vi "fpga_8ch_Timestamping_BaselineCh_ov_debug.vi"(0 "Main clock":u32, 1 "Scheduler":u8, 2 "Baseline Ch":u8, 3 "Signal IN":T2, 4 "overflow":bool) -> (5 "Data available":T2, 6 "Timeouts Bundle":T1, 7 "Timestamp bundle":T3)   [LabVIEW 2011]
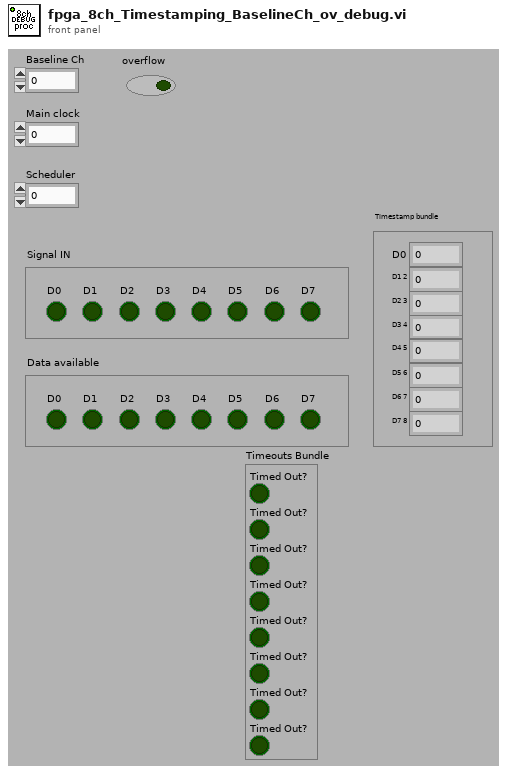
[diagram p1: front panel]
types:
  T1 = cluster{"Timed Out?":bool, "Timed Out?":bool, "Timed Out?":bool, "Timed Out?":bool, "Timed Out?":bool, "Timed Out?":bool, "Timed Out?":bool, "Timed Out?":bool}
  T2 = cluster{"D0":bool, "D1":bool, "D2":bool, "D3":bool, "D4":bool, "D5":bool, "D6":bool, "D7":bool}
  T3 = cluster{"D0":u32, "D1 2":u32, "D2 3":u32, "D3 4":u32, "D4 5":u32, "D5 6":u32, "D6 7":u32, "D7 8":u32}
  T4 = cluster{"Data Available":bool, "Data Available":bool, "Data Available":bool, "Data Available":bool, "Data Available":bool, "Data Available":bool, "Data Available":bool, "Data Available":bool}
  T5 = cluster{"32 bit Output":u32, "32 bit Output":u32, "32 bit Output":u32, "32 bit Output":u32, "32 bit Output":u32, "32 bit Output":u32, "32 bit Output":u32, "32 bit Output":u32}
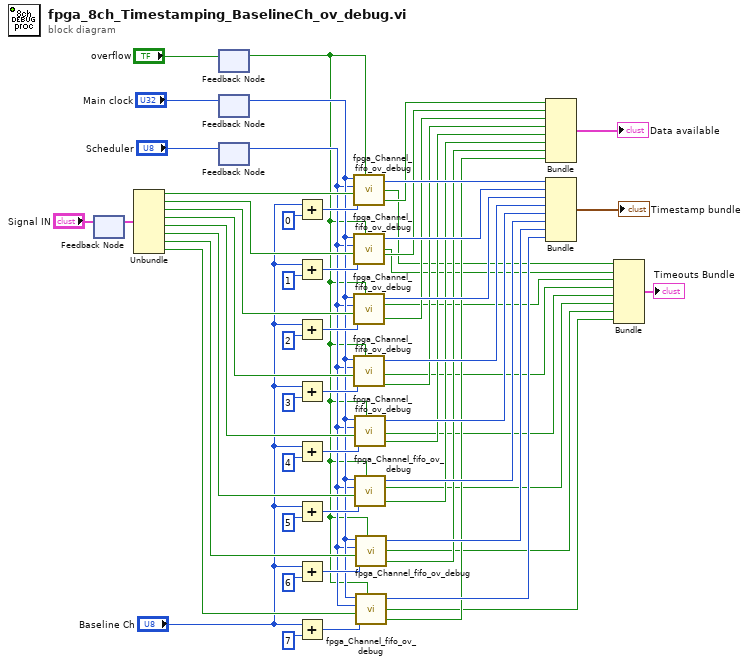
[diagram p0: block diagram]
diagram:
  n1 = feedback-in #1("Signal IN") -> ()
  n2 = feedback #1() -> (w12:T2)  [unwired: 1 in]
  n3 = Unbundle(w12) -> ("D0"=w59:bool, "D1"=w58:bool, "D2"=w57:bool, "D3"=w56:bool, "D4"=w55:bool, "D5"=w54:bool, "D6"=w53:bool, "D7"=w52:bool)
  n4 = feedback #2() -> (w10:bool)  [unwired: 1 in]
  n5 = feedback-in #2("overflow") -> ()
  n6 = feedback-in #3("Main clock") -> ()
  n7 = feedback #3() -> (w15:u32)  [unwired: 1 in]
  n8 = feedback #4() -> (w13:u8)  [unwired: 1 in]
  n9 = feedback-in #4("Scheduler") -> ()
  n10 = Add(x="Baseline Ch", y=u8 0 ("ID")) -> (x+y=w32:u8)
  n11 = Add(x="Baseline Ch", y=u8 1 ("ID")) -> (x+y=w19:u8)
  n12 = Add(x="Baseline Ch", y=u8 2 ("ID")) -> (x+y=w20:u8)
  n13 = Add(x="Baseline Ch", y=u8 3 ("ID")) -> (x+y=w17:u8)
  n14 = Add(x="Baseline Ch", y=u8 4 ("ID")) -> (x+y=w21:u8)
  n15 = Add(x="Baseline Ch", y=u8 5 ("ID")) -> (x+y=w22:u8)
  n16 = Add(x="Baseline Ch", y=u8 6 ("ID")) -> (x+y=w23:u8)
  n17 = Add(x="Baseline Ch", y=u8 7 ("ID")) -> (x+y=w24:u8)
  n18 = call "fpga_Channel_fifo_ov_debug.vi"("Main clock"=w15, "Scheduler"=w13, "Signal IN"=w59, "ID"=w32, "overflow"=w10) -> ("32 bit Output"=w51:u32, "Timed Out?"=w9:bool, "Data Available"=w42:bool)
  n19 = call "fpga_Channel_fifo_ov_debug.vi"("Main clock"=w15, "Scheduler"=w13, "Signal IN"=w58, "ID"=w19, "overflow"=w10) -> ("32 bit Output"=w50:u32, "Timed Out?"=w8:bool, "Data Available"=w41:bool)
  n20 = call "fpga_Channel_fifo_ov_debug.vi"("Main clock"=w15, "Scheduler"=w13, "Signal IN"=w57, "ID"=w20, "overflow"=w10) -> ("32 bit Output"=w49:u32, "Timed Out?"=w7:bool, "Data Available"=w40:bool)
  n21 = call "fpga_Channel_fifo_ov_debug.vi"("Main clock"=w15, "Scheduler"=w13, "Signal IN"=w56, "ID"=w17, "overflow"=w10) -> ("32 bit Output"=w48:u32, "Timed Out?"=w6:bool, "Data Available"=w39:bool)
  n22 = call "fpga_Channel_fifo_ov_debug.vi"("Main clock"=w15, "Scheduler"=w13, "Signal IN"=w55, "ID"=w21, "overflow"=w10) -> ("32 bit Output"=w47:u32, "Timed Out?"=w5:bool, "Data Available"=w38:bool)
  n23 = call "fpga_Channel_fifo_ov_debug.vi"("Main clock"=w15, "Scheduler"=w13, "Signal IN"=w54, "ID"=w22, "overflow"=w10) -> ("32 bit Output"=w46:u32, "Timed Out?"=w4:bool, "Data Available"=w37:bool)
  n24 = call "fpga_Channel_fifo_ov_debug.vi"("Main clock"=w15, "Scheduler"=w13, "Signal IN"=w53, "ID"=w23, "overflow"=w10) -> ("32 bit Output"=w45:u32, "Timed Out?"=w3:bool, "Data Available"=w36:bool)
  n25 = call "fpga_Channel_fifo_ov_debug.vi"("Main clock"=w15, "Scheduler"=w13, "Signal IN"=w52, "ID"=w24, "overflow"=w10) -> ("32 bit Output"=w44:u32, "Timed Out?"=w2:bool, "Data Available"=w35:bool)
  n26 = Bundle("Data Available"=w42, "Data Available"=w41, "Data Available"=w40, "Data Available"=w39, "Data Available"=w38, "Data Available"=w37, "Data Available"=w36, "Data Available"=w35) -> (→"Data available":T4)  [unwired: 1 in]
  n27 = Bundle("32 bit Output"=w51, "32 bit Output"=w50, "32 bit Output"=w49, "32 bit Output"=w48, "32 bit Output"=w47, "32 bit Output"=w46, "32 bit Output"=w45, "32 bit Output"=w44) -> (→"Timestamp bundle":T5)  [unwired: 1 in]
  n28 = Bundle("Timed Out?"=w9, "Timed Out?"=w8, "Timed Out?"=w7, "Timed Out?"=w6, "Timed Out?"=w5, "Timed Out?"=w4, "Timed Out?"=w3, "Timed Out?"=w2) -> (→"Timeouts Bundle":T1)  [unwired: 1 in]
